vi "Connect.vi"(8 "error in (no error)":errorcluster, 11 "Ultimus V in":refnum<class "Ultimus V.lvclass">) -> (0 "error out":errorcluster, 3 "Ultimus V out":refnum<class "Ultimus V.lvclass">)   [LabVIEW 2020, in "Ultimus V.lvclass"]
uses:
  Ultimus V.lvclass
  Ultimus V.lvclass/Ultimus V.ctl
  EFD Ultimus V/EFD Ultimus V.lvlib
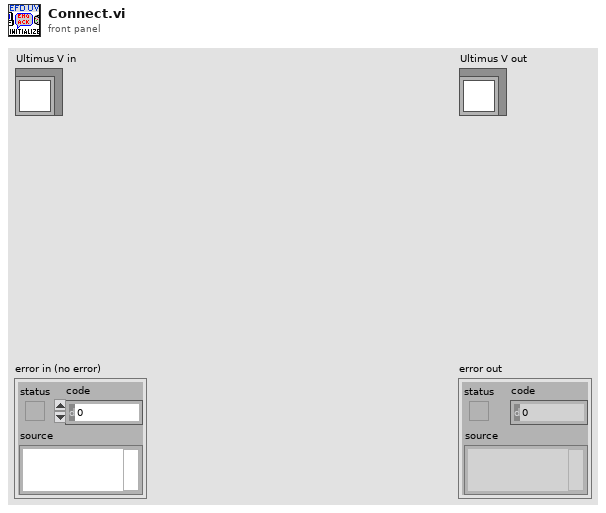
[diagram p1: front panel]
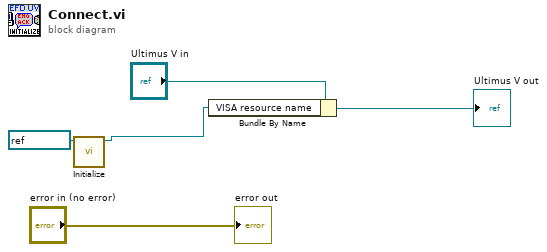
[diagram p0: block diagram]
diagram:
  n1 = call "Initialize.vi"("VISA resource name"=refnum<visa-resource-name> "COM1") -> ("VISA resource name out"=w2:refnum<visa-resource-name>)  [unwired: 8 in, 1 out]
  n2 = Bundle By Name(cluster="Ultimus V in", "VISA resource name"=w2) -> (→"Ultimus V out":refnum<class "Ultimus V.lvclass">)
  "error out" <- "error in (no error)"
